vi "Get Variables.vi"(8 "error in (no error)":errorcluster, 11 "Message Popup in":refnum<class "Assignment Statement.lvclass">) -> (0 "error out":errorcluster, 2 "Variables":variant, 3 "Message Popup out":refnum<class "Assignment Statement.lvclass">)   [LabVIEW 2016, in "Assignment Statement.lvclass"]
uses:
  Assignment Statement.lvclass
  Assignment Statement.lvclass/Assignment Statement.ctl
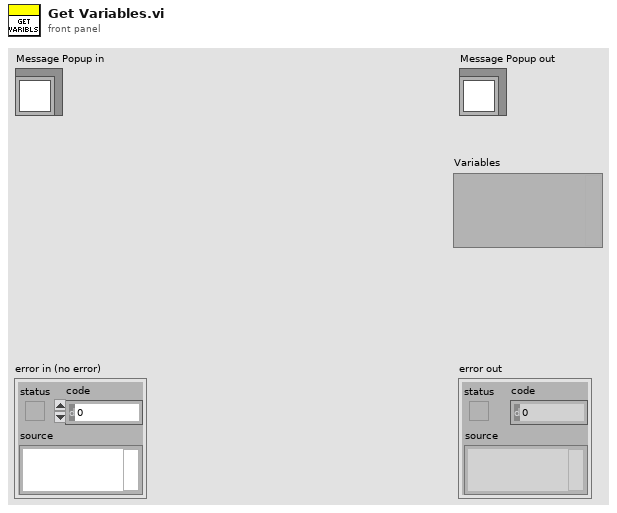
[diagram p1: front panel]
types:
  T1 = typedef "Assignment Statement.lvclass/Variables.ctl" = cluster{"leftoperand":string, "rightoperand":variant}
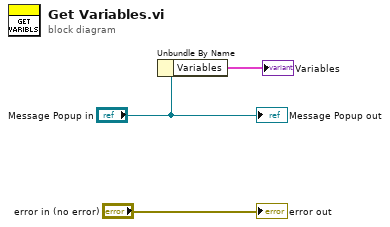
[diagram p0: block diagram]
diagram:
  n1 = Unbundle By Name("Message Popup in") -> ("Variables"=→"Variables":T1)
  "error out" <- "error in (no error)"
  "Message Popup out" <- "Message Popup in"
